vi "Hide Windows Taskbar.vi"(4 "error in (no error)":errorcluster, 7 "Operation":u16(ring) items=["Hide Taskbar", "Unhide Taskbar"]) -> (0 "error out":errorcluster)   [LabVIEW 2014, in "Master.lvclass"]
doc: "The Hide Windows Taskbar VI will programmatically show or hide the Windows Taskbar. This can be useful if you need to use the full screen of the primary monitor and not allow the user access to the Start Menu with the mouse. Press <Ctrl-Esc> to show the Start Menu.\n\nThe VI calls the Windows API and uses the SetWindowPos function.\n\nOpen and run the Test HWT VI to demonstrate the functionality of the Hide Windows Taskbar VI."
uses:
  Master/Master.lvclass
  user32.dll
panel:
  # "Select Help»Show Context Help and move the cursor over the VI icon to display help for this VI."
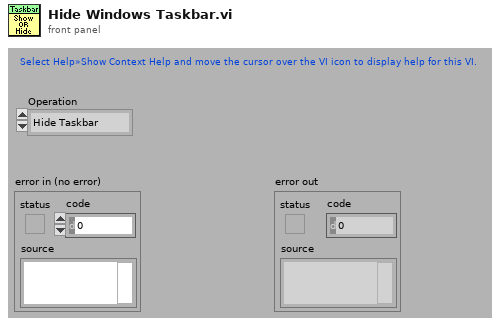
[diagram p1: front panel]
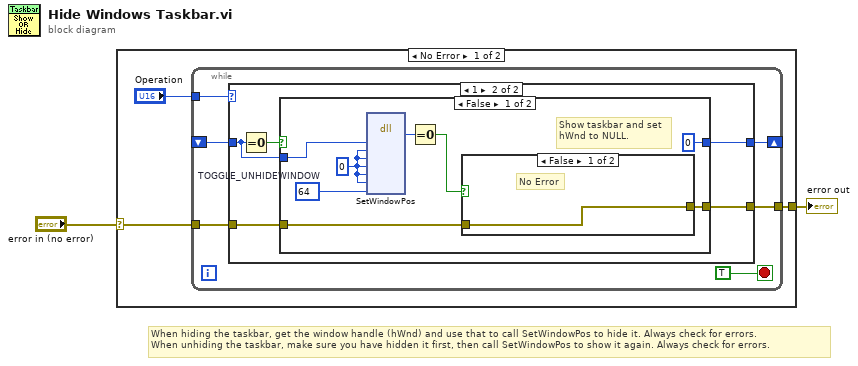
[diagram p0: block diagram]
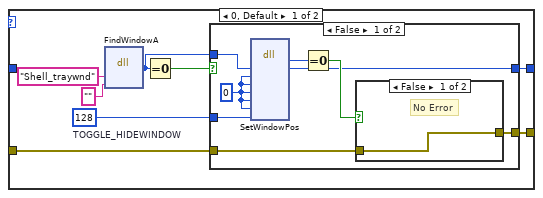
[diagram p2: hidden frame]
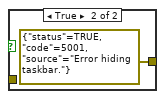
[diagram p3: hidden frame]
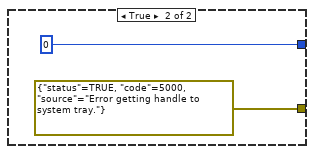
[diagram p4: hidden frame]
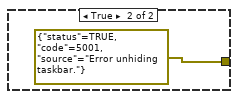
[diagram p5: hidden frame]
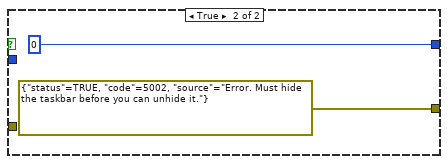
[diagram p6: hidden frame]
diagram:
  # "When hiding the taskbar, get the window handle (hWnd) and use that to call SetWindowPos to hide it. Always check for errors.\nWhen unhiding the taskbar, make sure you have hidden it first, then call SetWindowPos to show it again. Always check for errors."
  n1 = case shown="No Error" "error in (no error)" {
    selector: "error in (no error)" -> [w3 w49]
    tunnel: [w4 w49] -> w2
    frame No Error {
      n2 = while {
        shift-right: [w10] -> _
        shift-left: _ -> [w9]
        tunnel: "Operation" -> [w11]
        tunnel: [w8] -> w4
        tunnel: w3 -> [w7]
        stop <- TRUE stop-if-true
        n3 = case shown="1" w11 {
          tunnel: [w16 w36] -> w10
          tunnel: w9 -> [_ w34]
          tunnel: [w13 w32] -> w8
          tunnel: w7 -> [w12 w33]
          frame 0, Default {
            w17 = u32 128  # TOGGLE_HIDEWINDOW
            n4 = dll-call lib="USER32.DLL" fn="FindWindowA"("lpClassName"="Shell_traywnd", "lpWindowName"="") -> ("hWnd"=w14:i32)  [unwired: 5 in, 2 out]
            n5 = Equal To 0?(x=w14) -> (x = 0?=w15:bool)
            n6 = case shown="False" w15 {
              tunnel: w17 -> [w27 _]
              tunnel: [w20 0 ("hWnd")] -> w16
              tunnel: w14 -> [w25 _]
              tunnel: [w22 errorcluster {"status"=TRUE, "code"=5000, "source"="Error getting handle to system tray."} ("error out")] -> w13
              tunnel: w12 -> [w21 _]
              frame False {
                w26 = 0
                n7 = dll-call lib="USER32.DLL" fn="SetWindowPos"("hWnd"=w25, "hWndInsertAfter"=w26, "X"=w26, "Y"=w26, "cx"=w26, "cy"=w26, "uFlags"=w27) -> ("bool"=w24:i32, "hWnd"=w20:i32)  [unwired: 9 in, 2 out]
                n8 = Equal To 0?(x=w24) -> (x = 0?=w23:bool)
                n9 = case shown="False" w23 {
                  tunnel: [w28 errorcluster {"status"=TRUE, "code"=5001, "source"="Error hiding taskbar."} ("error out")] -> w22
                  tunnel: w21 -> [w28 _]
                  frame False {
                    # "No Error"
                  }
                  frame True {
                  }
                }
              }
              frame True {
              }
            }
          }
          frame 1 {
            n10 = Equal To 0?(x=w34) -> (x = 0?=w35:bool)
            n11 = case shown="False" w35 {
              tunnel: [0 ("hWnd") 0 ("hWnd")] -> w36
              tunnel: w34 -> [w42 _]
              tunnel: w33 -> [w39 _]
              tunnel: [w38 errorcluster {"status"=TRUE, "code"=5002, "source"="Error. Must hide the taskbar before you can unhide it."} ("error out")] -> w32
              frame False {
                w43 = 0
                w44 = u32 64  # TOGGLE_UNHIDEWINDOW
                # "Show taskbar and set\nhWnd to NULL."
                n12 = dll-call lib="USER32.DLL" fn="SetWindowPos"("hWnd"=w42, "hWndInsertAfter"=w43, "X"=w43, "Y"=w43, "cx"=w43, "cy"=w43, "uFlags"=w44) -> ("bool"=w41:i32)  [unwired: 10 in, 2 out]
                n13 = Equal To 0?(x=w41) -> (x = 0?=w40:bool)
                n14 = case shown="False" w40 {
                  tunnel: [w45 errorcluster {"status"=TRUE, "code"=5001, "source"="Error unhiding taskbar."} ("error out")] -> w38
                  tunnel: w39 -> [w45 _]
                  frame False {
                    # "No Error"
                  }
                  frame True {
                  }
                }
              }
              frame True {
              }
            }
          }
        }
      }
    }
    frame Error {
      # "Previous Error. Pass it through."
    }
  }
  "error out" <- w2
